vi "Send Command.vi"(8 "error in (no error)":errorcluster, 10 "command":string, 11 "VISA resource name":refnum<visa-resource-name>="COM1") -> (0 "error out":errorcluster, 3 "VISA resource name out":refnum<visa-resource-name>)   [LabVIEW 2017]
panel:
  out "read buffer":string
  in  "byte count":u32=8
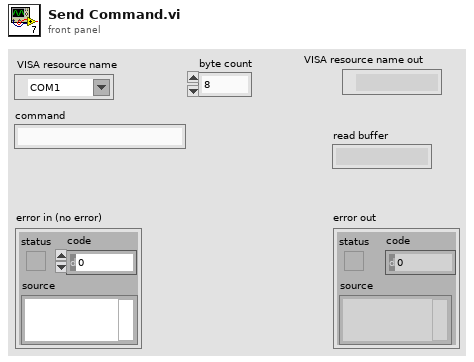
[diagram p1: front panel]
types:
  T1 = typedef "Semaphore RefNum" = refnum<k1>
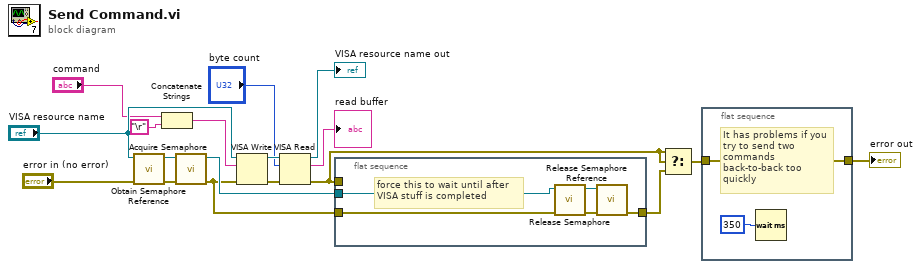
[diagram p0: block diagram]
diagram:
  n1 = call <vilib>:"Obtain Semaphore Reference.vi"("error in (no error)"="error in (no error)", "name (unnamed)"="VISA resource name") -> ("error out"=w17:errorcluster, "semaphore"=w18:T1)  [unwired: 1 in, 3 out]
  n2 = Concatenate Strings("command", "\r") -> (w1:string)
  n3 = call <vilib>:"Acquire Semaphore.vi"("error in (no error)"=w17, "semaphore"=w18) -> ("error out"=w13:errorcluster, "semaphore out"=w15:T1)  [unwired: 1 in, 3 out]
  n4 = VISA Write(VISA resource name="VISA resource name", write buffer=w1, error in (no error)=w13) -> (VISA resource name out=w11:refnum<visa-resource-name>, error out=w9:errorcluster)  [unwired: 1 out]
  n5 = VISA Read(VISA resource name=w11, byte count="byte count", error in (no error)=w9) -> (VISA resource name out=→"VISA resource name out":refnum<visa-resource-name>, read buffer=→"read buffer":string, error out=w8:errorcluster)  [unwired: 1 out]
  n6 = flat-sequence {
    tunnel: w15 -> [w23]
    tunnel: [w20] -> w12
    tunnel: w8 -> [_]
    tunnel: w13 -> [w19]
    frame #0 {
      # "force this to wait until after \nVISA stuff is completed"
      n7 = call <vilib>:"Release Semaphore.vi"("error in (no error)"=w19, "semaphore"=w23) -> ("error out"=w21:errorcluster, "semaphore out"=w22:T1)  [unwired: 4 out]
      n8 = call <vilib>:"Release Semaphore Reference.vi"("error in (no error)"=w21, "semaphore"=w22) -> ("error out"=w20:errorcluster)  [unwired: 9 out]
    }
  }
  n9 = Select(t=w8, s=w8, f=w12) -> (s? t:f=w5:errorcluster)
  n10 = flat-sequence {
    tunnel: w5 -> [w25]
    tunnel: [w25] -> w4
    frame #0 {
      # "It has problems if you try to send two commands back-to-back too quickly"
      n11 = Wait (ms)(milliseconds to wait=u32 350) -> ()  [unwired: 1 out]
    }
  }
  "error out" <- w4
